vi "main_0_1.vi"() -> ()   [LabVIEW 2013]
uses:
  sub vi/imaging/Image.ctl
  sub vi/gui event/GUI control.ctl
  sub vi/init & communication/Setting-User input.ctl
  <vilib>/Utility/error.llb/DialogType.ctl
  sub vi/imaging/Imaging State.ctl
  sub vi/init & communication/event-package.ctl
  sub vi/init & communication/Event1.ctl
  <vilib>/Utility/error.llb/Error Cluster From Error Code.vi
  <vilib>/Utility/file.llb/Write To Spreadsheet File (DBL).vi
  <vilib>/ErrorRing/Error Ring.xnode
panel:
  in  "Setting User Input":T1 {"Zoom (V)" scale=0.0..1.0; "X Pos." scale=-2.0..2.0; "Y Pos." scale=-2.0..2.0}
  in  "Event Controls":T2={"stop"=FALSE, "save sheet"=FALSE, "Path"=path "D:/Zhiping/ScanImage-LabVIEW/data/20170319_02.tif", "save tiff"=FALSE, "Gain"=150.0, "Offset"=0.0} {"Offset" scale=-1.0..1.0; "Gain" scale=0.0..150.0}
  out "Image":T3
  # "选取并移动游标至需要成像的\n中心位置后，会自动设置对应\n的x、y方向中心电压。再次运\n行程序，即可以上次选取的位\n置为中心成像。"
  # "使用步骤：\n\n1. 设置Setting User Input中的项目。\n2. 运行程序。\n3. 运行时可以调节图像游标、增益、偏置以及文件保存地址，\n    以及使用保存功能。\n\n（\"ctrl+h\"打开快捷帮助后，鼠标悬停可见各控件的具体帮助）"
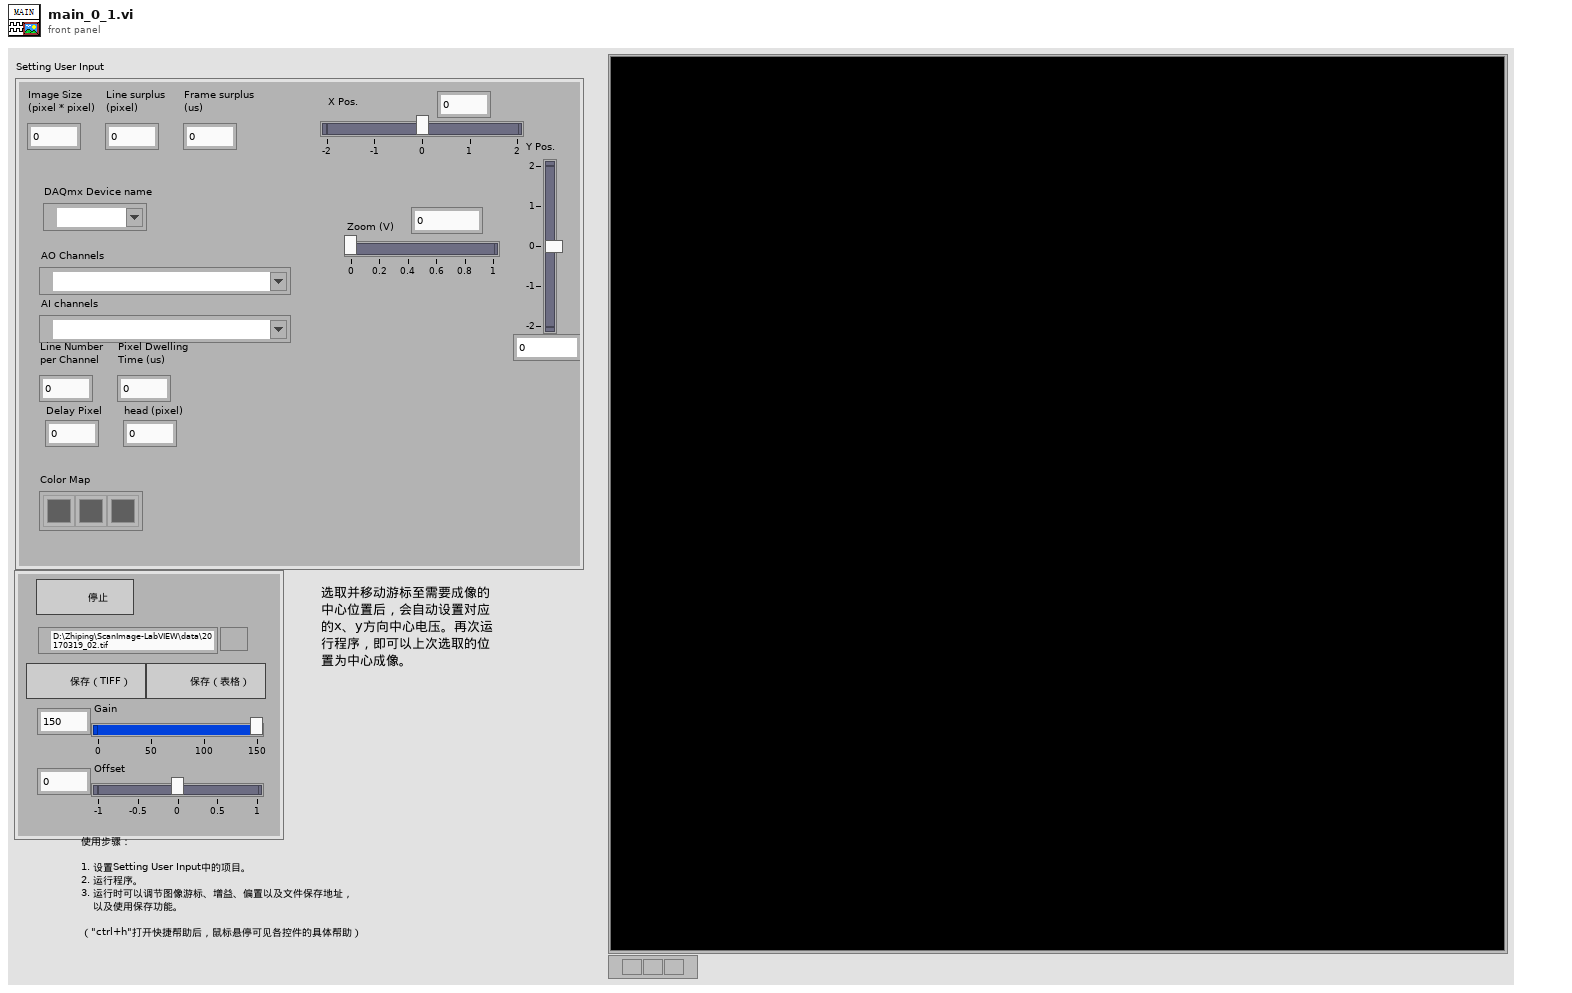
[diagram p1: front panel]
types:
  T1 = typedef "Setting-User input.ctl" = cluster{"Image Size\n(pixel * pixel)":i32, "AO Channels":tag, "Y Pos.":dbl, "X Pos.":dbl, "Line surplus\n(pixel)":i32, "Frame surplus\n(us)":i32, "AI channels":tag, "Line Number\nper Channel":i32, "Delay Pixel":i32, "Pixel Dwelling\nTime (us)":i32, "Color Map":u32[], "head (pixel)":i32, "Zoom (V)":dbl, "DAQmx Device name":tag}
  T2 = typedef "GUI control.ctl" = cluster{"stop":bool, "save sheet":bool, "Path":path, "save tiff":bool, "Gain":dbl, "Offset":dbl}
  T3 = typedef "Image.ctl" = dbl[][]
  T4 = typedef "Imaging State.ctl" = enum16{"idle", "waiting for saving sheet", "waiting for stopping", "waiting for saving tiff", "initial"}
  T5 = typedef "DialogType.ctl" = u16
  T6 = typedef "init-status.ctl" = cluster{"Setting":T7, "Event Queue":refnum<queue>, "Data Queue":refnum<queue>, "rendezvous":T8, "CO task out":refnum<k21>, "AO task out":refnum<k21>, "AI task out":refnum<k21>}
  T7 = typedef "Setting.ctl" = cluster{"Image Size\n(pixel * pixel)":i32, "Counter Channel":tag, "Trigger Term":tag, "AO Channels":tag, "Y Pos.":cluster{dbl, dbl}, "X Pos.":cluster{dbl, dbl}, "Line surplus\n(pixel)":i32, "Frame surplus\n(us)":i32, "AI channels":tag, "Line Number\nper Channel":i32, "Delay Pixel":i32, "Pixel Dwelling\nTime (us)":i32, "Color Map":u32[], "head (pixel)":i32}
  T8 = typedef "Rendezvous RefNum" = refnum<k1>
  T9 = typedef "event-package.ctl" = cluster{"Event":T10, "Data":string}
  T10 = typedef "Event1.ctl" = enum16{"null", "stop AI", "stop AO", "stop Imaging", "stop Counter", "save sheet", "restart", "save tiff", "gain/offset changed"}
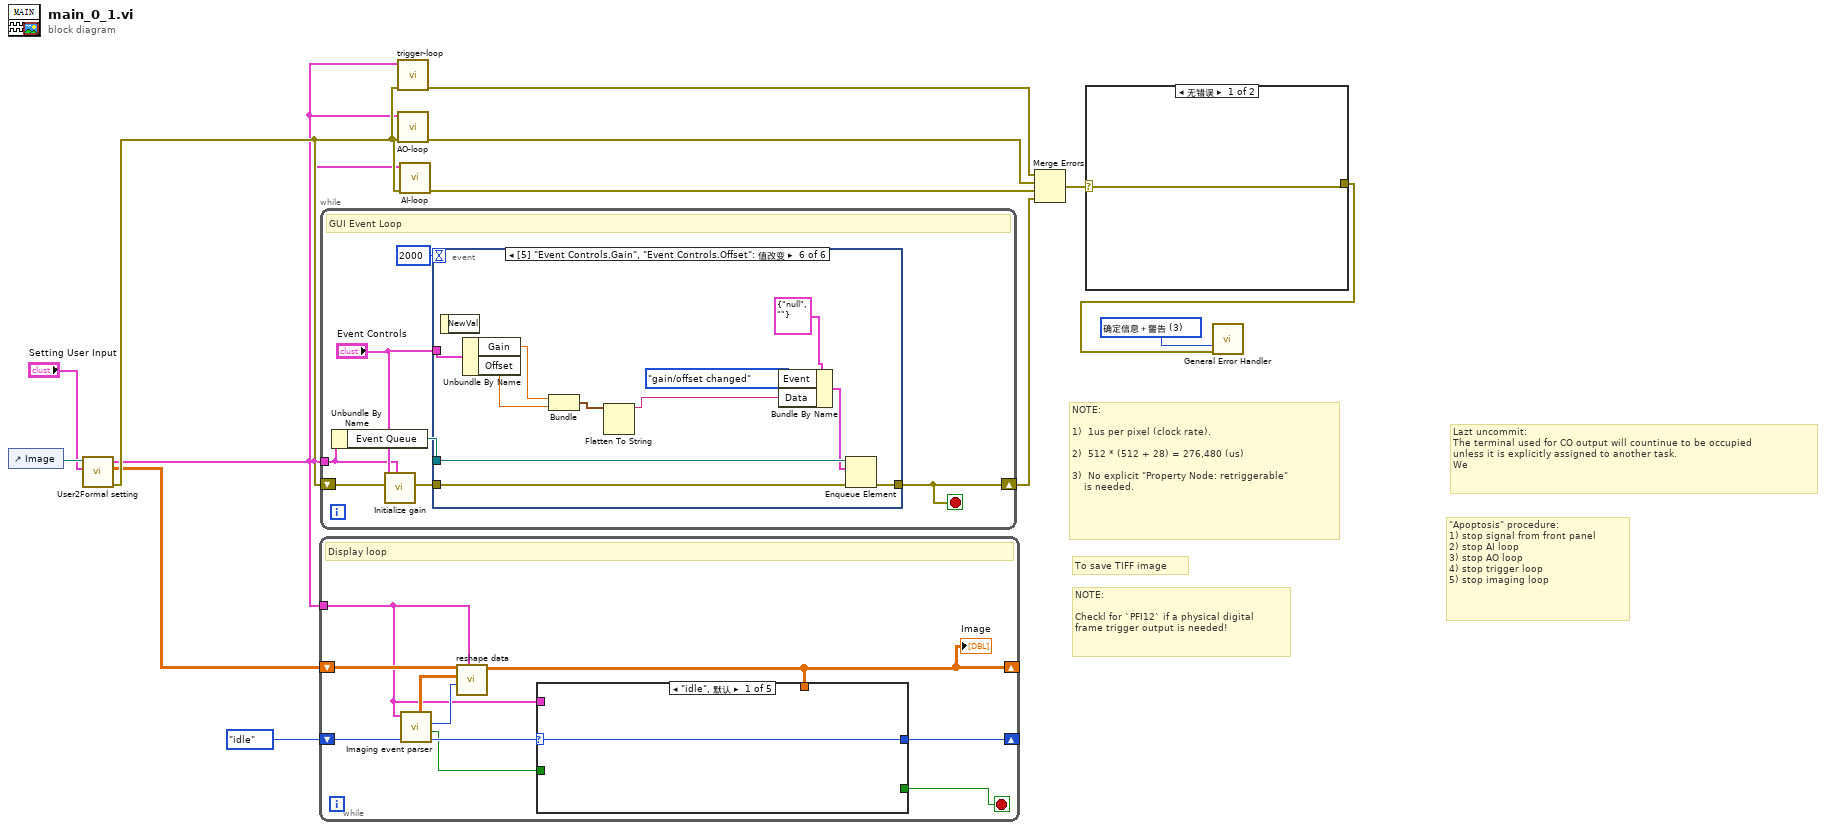
[diagram p0: block diagram]
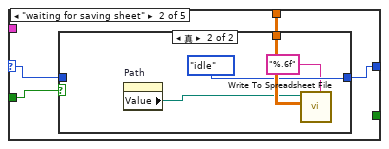
[diagram p2: hidden frame]
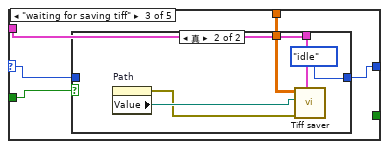
[diagram p4: hidden frame]
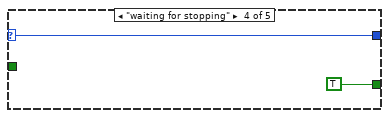
[diagram p6: hidden frame]
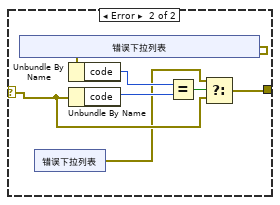
[diagram p8: hidden frame]
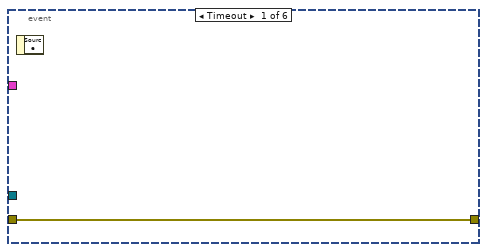
[diagram p9: hidden frame]
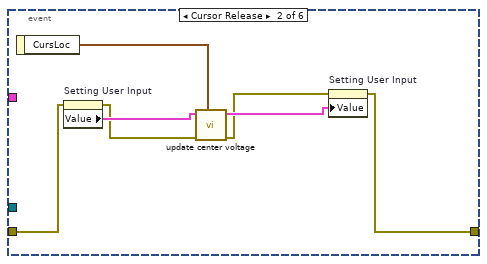
[diagram p10: hidden frame]
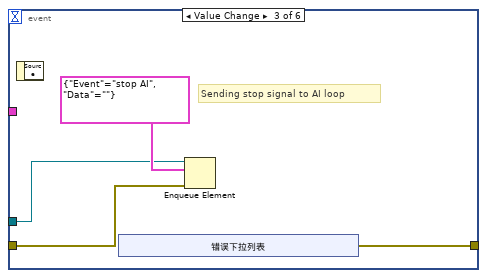
[diagram p11: hidden frame]
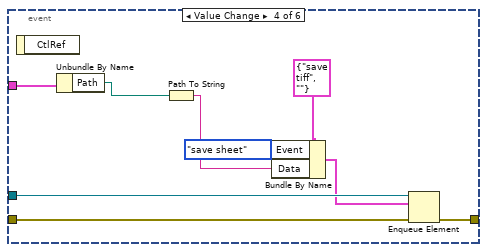
[diagram p12: hidden frame]
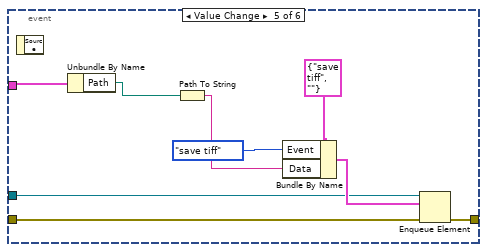
[diagram p13: hidden frame]
diagram:
  w8 = T5 3 items=["无对话框", "确定信息", "继续或停止信息", "确定信息＋警告", "继续/停止+警告"] ("type of dialog (OK msg:1)")
  # "To save TIFF image"
  # "Lazt uncommit:\nThe terminal used for CO output will countinue to be occupied\nunless it is explicitly assigned to another task.\nWe"
  # "\"Apoptosis\" procedure:\n1) stop signal from front panel\n2) stop AI loop\n3) stop AO loop\n4) stop trigger loop\n5) stop imaging loop"
  # "NOTE:\n\nCheckl for `PFI12` if a physical digital\nframe trigger output is needed!"
  # "NOTE:\n\n1)  1us per pixel (clock rate).\n\n2)  512 * (512 + 28) = 276,480 (us)\n\n3)  No explicit \"Property Node: retriggerable\"\n    is needed."
  n1 = control-ref of="Image"() -> (w2:refnum<vi>)
  n2 = call "User2Formal setting.vi"("Setting User Input"="Setting User Input", "IntensityGraph输入"=w2) -> ("错误输出"=w13:errorcluster, "Image 2"=w3:T3, "Status"=w5:T6)  [unwired: 7 in]
  n3 = while {
    tunnel: w5 -> [w14]
    shift-right: [w16] -> _
    shift-left: w3 -> [w18]
    shift-right: [w23] -> _
    shift-left: Imaging_State."idle" -> [w21]
    stop <- w22 stop-if-true
    # "Display loop"
    n4 = call "Imaging event parser.vi"("Imaging State in"=w21, "Status"=w14) -> ("Imaging State out"=w20:T4, "last line?"=w19:bool, "line #"=w17:i32, "Effective lines"=w15:dbl[][])  [unwired: 5 in, 1 out]
    n5 = call "reshape data.vi"("Status"=w14, "line #"=w17, "Effective lines"=w15, "Image输入"=w18) -> ("Image输出"=w16:T3)  [unwired: 7 in]
    "Image" <- w16
    n6 = case shown="\"idle\", 默认" w20 {
      selector: w20 -> [w24 w26 w36 w45 w47]
      tunnel: w16 -> [_ w28 w38 _ _]
      tunnel: [w24 w25 w35 w45 w47] -> w23
      tunnel: [_ _ _ TRUE _] -> w22
      tunnel: w19 -> [_ w27 w37 _ _]
      tunnel: w14 -> [_ _ w34 _ _]
      frame "idle", Default {
      }
      frame "waiting for saving sheet" {
        n7 = case shown="真" w27 {
          tunnel: w28 -> [_ w33]
          tunnel: w26 -> [w29 _]
          tunnel: [w29 Imaging_State."idle"] -> w25
          frame False {
          }
          frame True {
            n8 = property on="Path" class="Path"() -> ("Value"=w30:path)  [unwired: 2 in, 2 out]
            n9 = call-poly <vilib>:"Write To Spreadsheet File.vi"("format (%.3f)"="%.6f", "2D data"=w33, "file path (dialog if empty)"=w30) -> ()  [unwired: 5 in, 1 out]
          }
        }
      }
      frame "waiting for saving tiff" {
        n10 = case shown="真" w37 {
          tunnel: w38 -> [_ w40]
          tunnel: w36 -> [w39 _]
          tunnel: [w39 Imaging_State."idle"] -> w35
          tunnel: w34 -> [_ w41]
          frame False {
          }
          frame True {
            n11 = property on="Path" class="Path"() -> (error out=w42:errorcluster, "Value"=w43:path)  [unwired: 2 in, 1 out]
            n12 = call "Tiff saver.vi"("Status"=w41, "error in (no error)"=w42, "File Path"=w43, "Image in"=w40) -> ()  [unwired: 7 in, 1 out]
          }
        }
      }
      frame "waiting for stopping" {
      }
      frame "initial" {
      }
    }
  }
  n13 = while {
    tunnel: w5 -> [w48]
    shift-right: [w54] -> w12
    shift-left: w13 -> [w51]
    stop <- w54 stop-if-true
    # "GUI Event Loop"
    n14 = Unbundle By Name(w48) -> ("Event Queue"=w52:refnum<queue>)
    n15 = call "Initialize gain.vi"("Status"=w48, "错误输入（无错误）"=w51, "Event Controls"="Event Controls") -> ("error out"=w50:errorcluster)  [unwired: 8 in]
    n16 = event shown="[5] \"Event Controls.Gain\", \"Event Controls.Offset\": 值改变" {
      selector: _ -> [_ _ _ _ _ _]
      dyn-events: _ -> [_ _ _ _ _ _]
      timeout: 2000 -> [_ _ _ _ _ _]
      tunnel: w50 -> [w55 w56 w63 w78 w82 w96]
      tunnel: [w55 w57 w66 w77 w81 w95] -> w54
      tunnel: w52 -> [_ _ w64 w79 w83 w99]
      tunnel: "Event Controls" -> [_ _ _ w76 w80 w91]
      event Timeout {
        n17 = event-data() -> ()  [unwired: 1 in, 1 out]
      }
      event Cursor Release {
        n18 = event-data() -> ("CursLoc"=w61:cluster{"X":dbl, "Y":dbl})  [unwired: 1 in]
        n19 = property on="Setting User Input" class="Clust (严格)"(error in=w56) -> (error out=w59:errorcluster, "Value"=w60:T1)  [unwired: 1 in, 1 out]
        n20 = call "update center voltage.vi"("CursLoc"=w61, "错误输入（无错误）"=w59, "Value in"=w60) -> ("错误输出"=w58:errorcluster, "Value out"=w62:T1)  [unwired: 7 in]
        n21 = property on="Setting User Input" class="Clust (严格)"(error in=w58, "Value"=w62) -> (error out=w57:errorcluster)  [unwired: 1 in, 1 out]
      }
      event Value Change {
        # "Sending stop signal to AI loop"
        n22 = event-data() -> ()  [unwired: 1 in, 1 out]
        n23 = xnode "错误下拉列表"() -> ("错误输出"=w66:errorcluster)
        n24 = Enqueue Element(queue=w64, element=T9 {"Event"=enum."stop AI", "Data"=""} ("元素"), error in (no error)=w63) -> ()  [unwired: 1 in, 3 out]
      }
      event Value Change {
        n25 = event-data() -> ()  [unwired: 1 in, 1 out]
        n26 = Unbundle By Name(w76) -> ("Path"=w74:path)
        n27 = Path To String(path=w74) -> (string=w73:string)
        n28 = Bundle By Name(cluster=T9 {"Event"=enum."save tiff", "Data"=""} ("元素"), "Event"=Event1."save sheet", "Data"=w73) -> (w71:T9)
        n29 = Enqueue Element(queue=w79, element=w71, error in (no error)=w78) -> (error out=w77:errorcluster)  [unwired: 1 in, 2 out]
      }
      event Value Change {
        n30 = event-data() -> ()  [unwired: 1 in, 1 out]
        n31 = Unbundle By Name(w80) -> ("Path"=w87:path)
        n32 = Path To String(path=w87) -> (string=w86:string)
        n33 = Bundle By Name(cluster=T9 {"Event"=enum."save tiff", "Data"=""} ("元素"), "Event"=Event1."save tiff", "Data"=w86) -> (w84:T9)
        n34 = Enqueue Element(queue=w83, element=w84, error in (no error)=w82) -> (error out=w81:errorcluster)  [unwired: 1 in, 2 out]
      }
      event Value Change {
        n35 = event-data() -> ()  [unwired: 1 in, 1 out]
        n36 = Unbundle By Name(w91) -> ("Gain"=w90:dbl, "Offset"=w89:dbl)
        n37 = Bundle("Gain"=w90, "Offset"=w89) -> (w92:cluster{"Gain":dbl, "Offset":dbl})  [unwired: 1 in]
        n38 = Flatten To String(anything=w92) -> (data string=w93:string)  [unwired: 3 in, 2 out]
        n39 = Bundle By Name(cluster=T9 {"Event"=enum."null", "Data"=""} ("Event Package"), "Event"=Event1."gain/offset changed", "Data"=w93) -> (w94:T9)
        n40 = Enqueue Element(queue=w99, element=w94, error in (no error)=w96) -> (error out=w95:errorcluster)  [unwired: 1 in, 2 out]
      }
    }
  }
  n41 = call "trigger-loop.vi"("错误输入（无错误）"=w13, "Status"=w5) -> ("error out"=w11:errorcluster)  [unwired: 9 in]
  n42 = call "AO-loop.vi"("错误输入（无错误）"=w13, "Status"=w5) -> ("Error out"=w10:errorcluster)  [unwired: 9 in]
  n43 = call "AI-loop.vi"("错误输入（无错误）"=w13, "Status"=w5) -> ("Error out"=w9:errorcluster)  [unwired: 9 in]
  n44 = Merge Errors(w11, w10, w9, w12) -> (w7:errorcluster)
  n45 = case shown="无错误" w7 {
    selector: w7 -> [w100 w103]
    tunnel: [w100 w101] -> w6
    frame No Error {
    }
    frame Error {
      n46 = xnode "错误下拉列表"() -> ("错误输出"=w106:errorcluster)
      n47 = xnode "错误下拉列表"() -> ("错误输出"=w102:errorcluster)
      n48 = Unbundle By Name(w106) -> ("code"=w105:i32)
      n49 = Unbundle By Name(w103) -> ("code"=w104:i32)
      n50 = Equal?(x=w105, y=w104) -> (x = y?=w107:bool)
      n51 = Select(t=w102, s=w107, f=w103) -> (s? t:f=w101:errorcluster)
    }
  }
  n52 = call <vilib>:"General Error Handler.vi"("type of dialog (OK msg:1)"=w8, "error in (no error)"=w6) -> ()  [unwired: 9 in, 5 out]
